vi "22-09-2020.vi"() -> ()   [LabVIEW 2020]
panel:
  out "Sum":i16
  out "String present or not (0,1)":i16[](array[numeric])
  out "String is present or not":bool[](array[boolean])
  in  "String":string
  out "total objects":i32
  out "String 4":string
  in  "String 3":string
  out "sorted array":dbl[](array[numeric])
  in  "Array":dbl[](array[numeric])
  out "String 2":string
  out "unsigned byte array 2":u8[](array[numeric])
  in  "Numeric":dbl format="%#_13g"
  out "unsigned byte array":u8[](array[numeric])
  in  "String":string
  # "String ASCII"
  # "Sort 1D Array"
  # "Sort String Array"
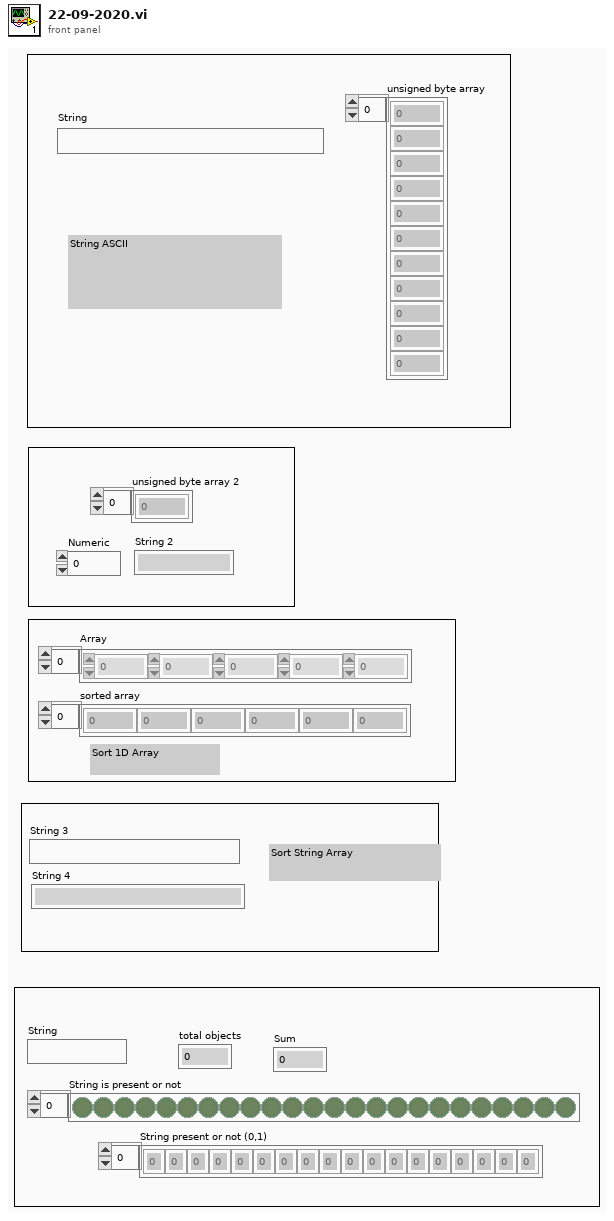
[diagram p1: front panel]
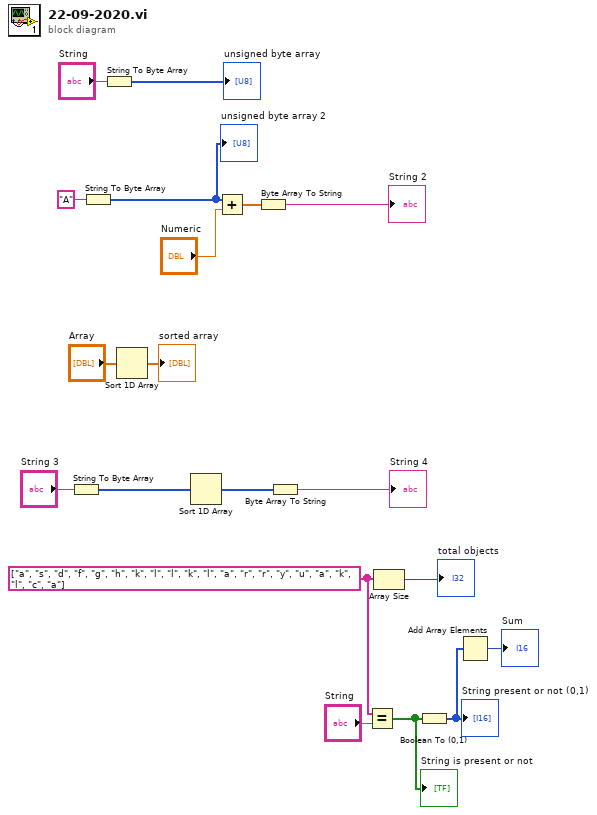
[diagram p0: block diagram]
diagram:
  w4 = string[] ["a", "s", "d", "f", "g", "h", "k", "l", "l", "k", "l", "a", "r", "r", "y", "u", "a", "k", "l", "c", "a"]
  n1 = String To Byte Array(string="String 3") -> (unsigned byte array=w9:u8[])
  n2 = String To Byte Array(string="A") -> (unsigned byte array=w15:u8[])
  "unsigned byte array 2" <- w15
  n3 = String To Byte Array(string="String") -> (unsigned byte array=→"unsigned byte array":u8[])
  n4 = Sort 1D Array(array="Array") -> (sorted array=→"sorted array":dbl[])
  n5 = Sort 1D Array(array=w9) -> (sorted array=w8:u8[])
  n6 = Add(x=w15, y="Numeric") -> (x+y=w14:dbl[])
  n7 = Byte Array To String(unsigned byte array=w14) -> (string=→"String 2":string)
  n8 = Byte Array To String(unsigned byte array=w8) -> (string=→"String 4":string)
  n9 = Equal?(x=w4, y="String") -> (x = y?=w3:bool[])
  "String is present or not" <- w3
  n10 = Array Size(array=w4) -> (size(s)=→"total objects":i32)
  n11 = Boolean To (0,1)(Boolean=w3) -> (0, 1=w2:i16[])
  "String present or not (0,1)" <- w2
  n12 = Add Array Elements(numeric array=w2) -> (sum=→"Sum":i16)
